vi "Write Output directory.vi"(8 "error in (no error)":errorcluster, 10 "Output directory":path, 11 "GObjectConverterBase in":refnum<class "GObjectConverterBase.lvclass">) -> (0 "error out":errorcluster, 3 "GObjectConverterBase out":refnum<class "GObjectConverterBase.lvclass">)   [LabVIEW 2017, in "GObjectConverterBase.lvclass"]
uses:
  GObjectConverterBase.lvclass
  GObjectConverterBase.lvclass/GObjectConverterBase.ctl
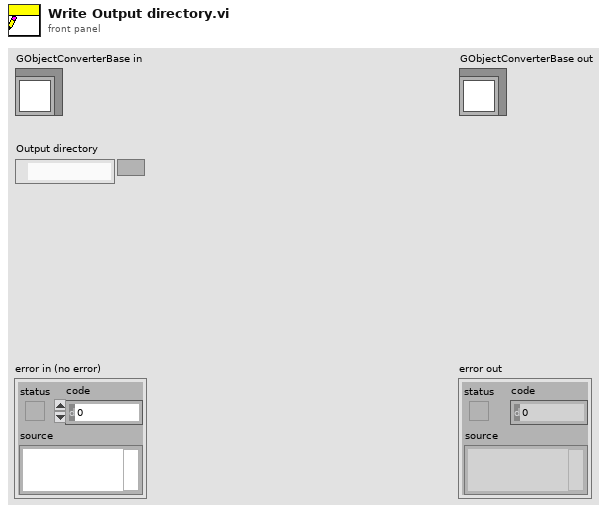
[diagram p1: front panel]
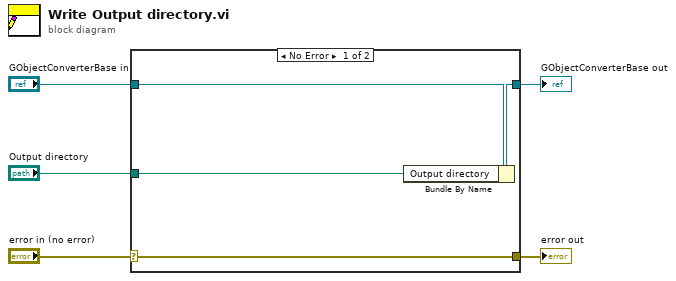
[diagram p0: block diagram]
diagram:
  n1 = case shown="No Error" "error in (no error)" {
    selector: "error in (no error)" -> [w9 w10]
    tunnel: [w9 w10] -> w4
    tunnel: [w7 w11] -> w2
    tunnel: "GObjectConverterBase in" -> [w8 w11]
    tunnel: "Output directory" -> [w6 _]
    frame No Error {
      n2 = Bundle By Name(cluster=w8, "Output directory"=w6) -> (w7:refnum<class "GObjectConverterBase.lvclass">)
    }
    frame Error {
    }
  }
  "error out" <- w4
  "GObjectConverterBase out" <- w2
